vi "Send GPIB commands.vi"(0 "Command list 1":T1(array[cluster]) {"Module" items=["Atom removal 1", "Atom removal 2", "B-field off", "CMOT", "Defaults", "Final B-field ramps", "Fluorescence pulse", "High field", "High field ARP", "Loading cart QT", "Loading sci QT", "Low field", "Low field ARP", "Mol OD image", "Mol picture", "Mol probe pulse", "Molasses", "MOT off", "MOT on", "OD image", "Optical pumping", "OT B-field off", "Picture", "Probe pulse", "QT off for OT", "Quadrupole trap off", "Quadrupole trap", "Quantization axis", "S-G separation", "STIRAP back for imaging", "STIRAP", "TTL high", "TTL low", "GPIB", "Utility Module 1", "Utility Module 2", "Utility Module 3", "Utility Module 4", "Utility Module 5", "Utility Module 6", "Utility Module 7", "Utility Module 8", "Utility Module 9"]; "Abs Start Time" format="%.3f"}, 1 "End time":dbl=83073.546, 2 "Abs start time":dbl=62269.999980926514, 3 "do it!":bool=TRUE) -> ()   [LabVIEW 2017]
doc: "This sends out GPIB commands during the experiment (after the DIO (TTL) board has been triggered."
uses:
  globals/Modules global.vi
panel:
  out "Array 2":dbl[](array[numeric])
  out "Array":string[](array[string])
  out "sorted array":T1(array[cluster])
  out "total time":dbl
  out "start time":dbl=3231522488.434
  in  "timeout ms":i32=1000
  out "error out":errorcluster
  # "enabled  time                                      GPIB address                       command"
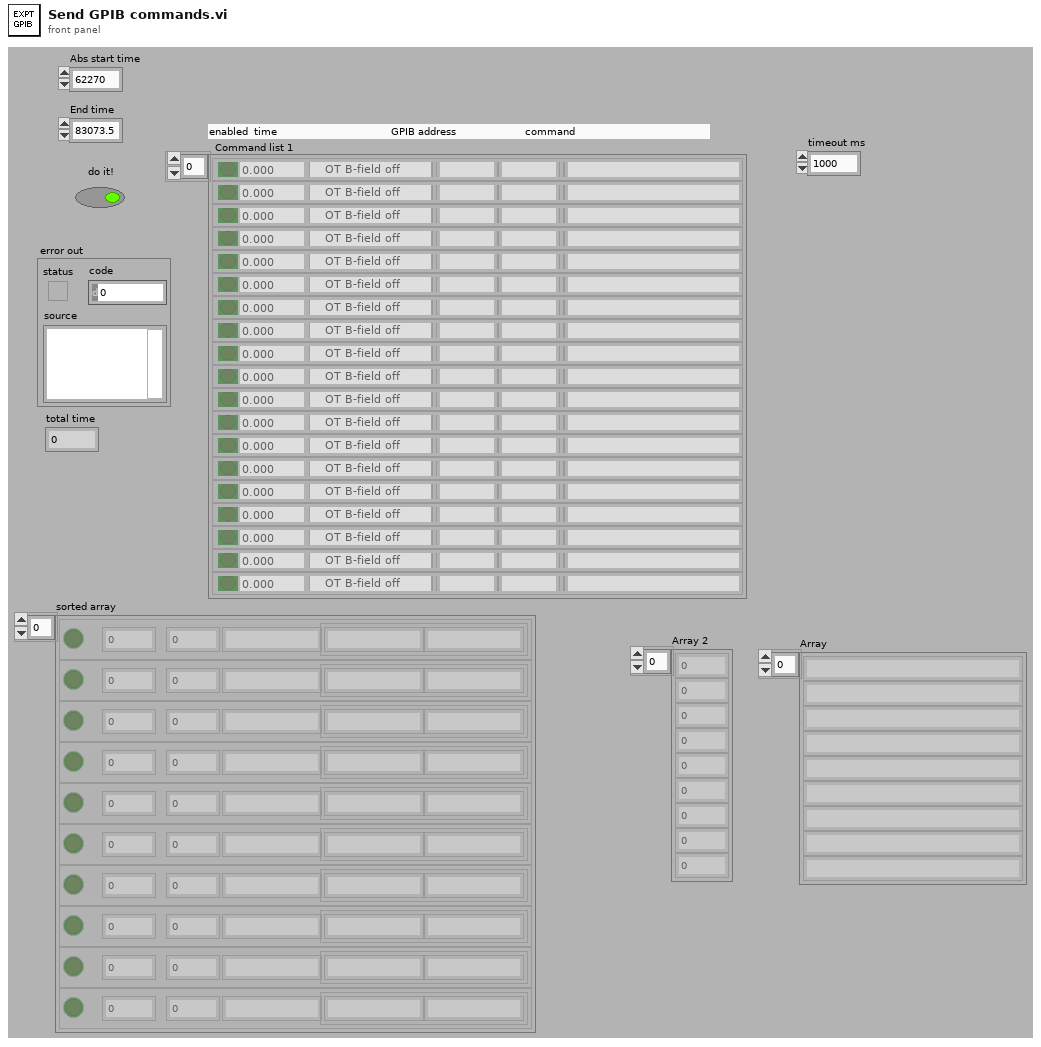
[diagram p1: front panel]
types:
  T1 = cluster{"Enable":bool, "Abs Start Time":dbl, "Module":u16, "String":string, "Array":string[]}[]
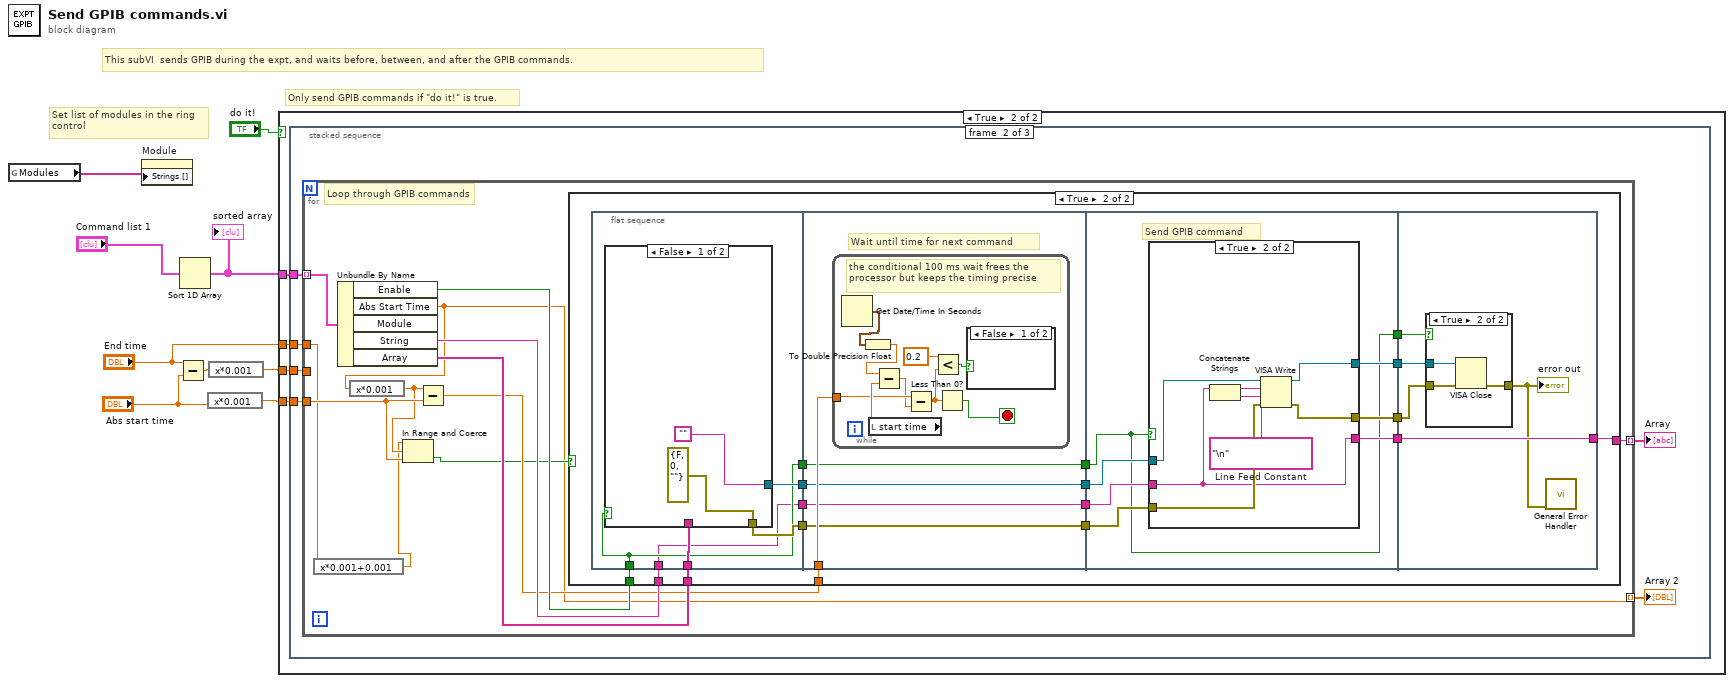
[diagram p0: block diagram]
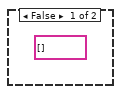
[diagram p2: hidden frame]
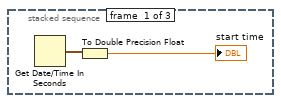
[diagram p3: hidden frame]
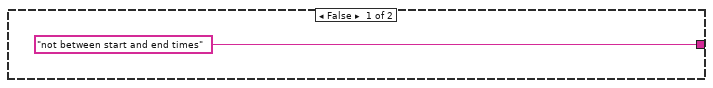
[diagram p4: hidden frame]
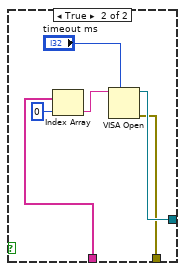
[diagram p5: hidden frame]
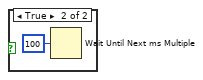
[diagram p6: hidden frame]
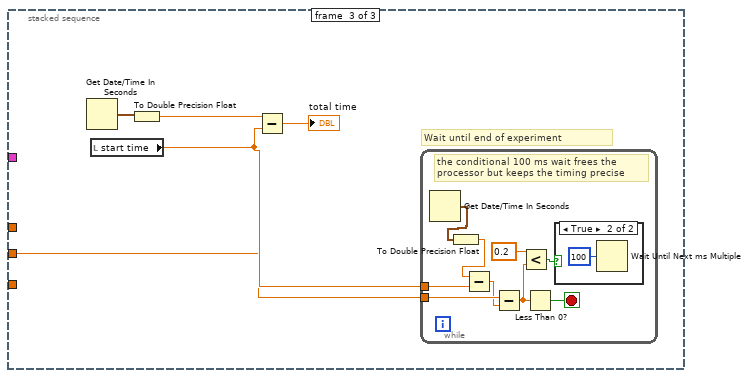
[diagram p9: hidden frame]
diagram:
  # "Set list of modules in the ring control"
  # "Only send GPIB commands if \"do it!\" is true."
  # "This subVI  sends GPIB during the expt, and waits before, between, and after the GPIB commands."
  n1 = global read "Modules global.vi" "Modules"() -> (w1:string[])
  n2 = property on="Module" class="Ring (strict)"("Strings []"=w1) -> ()  [unwired: 2 in, 2 out]
  n3 = Subtract(x="End time", y="Abs start time") -> (x-y=w8:dbl)
  n4 = Sort 1D Array(array="Command list 1") -> (sorted array=w3:T1)
  "sorted array" <- w3
  n5 = expression code="x*0.001"("Abs start time") -> (w5:dbl)
  n6 = expression code="x*0.001"(w8) -> (w7:dbl)
  n7 = case shown="True" "do it!" {
    tunnel: w5 -> [_ w13]
    tunnel: w7 -> [_ w12]
    tunnel: w3 -> [_ w11]
    tunnel: "End time" -> [_ w10]
    frame False {
      (unwired) string[] []
    }
    frame True {
      n8 = stacked-sequence {
        tunnel: w13 -> [_ w21 _]
        tunnel: w12 -> [_ w18 w106]
        tunnel: w11 -> [_ w20 _]
        tunnel: w10 -> [_ w17 _]
        frame #0 {
          n9 = Get Date/Time In Seconds() -> (seconds since 1Jan1904=w15:timestamp)
          n10 = To Double Precision Float(number=w15) -> (double precision float=→"start time":dbl)
        }
        frame #1 {
          n11 = for {
            tunnel: w20 -> [w33] mode=indexing
            tunnel: w21 -> [w27]
            tunnel: w18 -> [_]
            tunnel: [w26] -> w16 mode=indexing
            tunnel: [w22] -> w19 mode=indexing
            tunnel: w17 -> [w24]
            # "Loop through GPIB commands"
            n12 = expression code="x*0.001+0.001"(w24) -> (w23:dbl)
            n13 = Unbundle By Name(w33) -> ("Enable"=w30:bool, "Abs Start Time"=w22:dbl, "String"=w32:string, "Array"=w31:string[])  [unwired: 1 out]
            n14 = expression code="x*0.001"(w22) -> (w25:dbl)
            n15 = In Range and Coerce(upper limit=w23, x=w25, lower limit=w27) -> (In Range?=w28:bool)  [unwired: 1 out]
            n16 = Subtract(x=w25, y=w27) -> (x-y=w29:dbl)
            n17 = case shown="True" w28 {
              tunnel: w32 -> [_ w49]
              tunnel: w31 -> [_ w48]
              tunnel: w30 -> [_ w50]
              tunnel: w29 -> [_ w51]
              tunnel: ["not between start and end times" ("String") w36] -> w26
              frame False {
              }
              frame True {
                n18 = flat-sequence {
                  tunnel: w50 -> [w53]
                  tunnel: w49 -> [w52]
                  tunnel: w48 -> [w54]
                  tunnel: [w52] -> w47
                  tunnel: [w56] -> w46
                  tunnel: [w55] -> w45
                  tunnel: [w53] -> w44
                  tunnel: w51 -> [w69]
                  tunnel: w47 -> [w66]
                  tunnel: w46 -> [w67]
                  tunnel: w45 -> [w65]
                  tunnel: w44 -> [w68]
                  tunnel: [w68] -> w43
                  tunnel: [w67] -> w42
                  tunnel: [w66] -> w41
                  tunnel: [w65] -> w40
                  tunnel: w43 -> [w80]
                  tunnel: w42 -> [w84]
                  tunnel: w41 -> [w85]
                  tunnel: w40 -> [w86]
                  tunnel: [w83] -> w39
                  tunnel: [w82] -> w38
                  tunnel: [w81] -> w37
                  tunnel: [w80] -> w35
                  tunnel: w39 -> [w99]
                  tunnel: w38 -> [w100]
                  tunnel: w37 -> [w101]
                  tunnel: [w101] -> w36
                  tunnel: w35 -> [w98]
                  frame #0 {
                    n19 = case shown="False" w53 {
                      tunnel: ["" w61] -> w56
                      tunnel: [errorcluster {"status"=FALSE, "code"=0, "source"=""} ("VISA Error") w60] -> w55
                      tunnel: w54 -> [_ w59]
                      frame False {
                      }
                      frame True {
                        n20 = Index Array(array=w59, index=0) -> (element=w62:string)
                        n21 = VISA Open(timeout (0)="timeout ms", VISA resource name=w62) -> (VISA resource name=w61:refnum<visa-resource-name>, error out=w60:errorcluster)  [unwired: 3 in]
                      }
                    }
                  }
                  frame #1 {
                    # "Wait until time for next command"
                    n22 = while {
                      tunnel: w69 -> [w71]
                      stop <- w75 stop-if-true
                      # "the conditional 100 ms wait frees the processor but keeps the timing precise"
                      n23 = Get Date/Time In Seconds() -> (seconds since 1Jan1904=w74:timestamp)
                      n24 = To Double Precision Float(number=w74) -> (double precision float=w73:dbl)
                      n25 = local read "start time"() -> (w72:dbl)
                      n26 = Subtract(x=w73, y=w72) -> (x-y=w70:dbl)
                      n27 = Subtract(x=w71, y=w70) -> (x-y=w76:dbl)
                      n28 = Less?(x=0.2 ("y"), y=w76) -> (x < y?=w77:bool)
                      n29 = Less Than 0?(x=w76) -> (x < 0?=w75:bool)
                      n30 = case shown="False" w77 {
                        frame False {
                        }
                        frame True {
                          n31 = Wait Until Next ms Multiple(millisecond multiple=u32 100) -> ()  [unwired: 1 out]
                        }
                      }
                    }
                  }
                  frame #2 {
                    # "Send GPIB command"
                    n32 = case shown="True" w80 {
                      tunnel: w86 -> [w87 w95]
                      tunnel: w85 -> [w88 w92]
                      tunnel: w84 -> [w89 w96]
                      tunnel: [w89 w94] -> w83
                      tunnel: [w88 w92] -> w81
                      tunnel: [w87 w93] -> w82
                      frame False {
                      }
                      frame True {
                        w90 = "\n"  # Line Feed Constant
                        n33 = Concatenate Strings(w92, w90) -> (w91:string)
                        n34 = VISA Write(VISA resource name=w96, write buffer=w91, error in (no error)=w95) -> (VISA resource name out=w94:refnum<visa-resource-name>, error out=w93:errorcluster)  [unwired: 1 out]
                      }
                    }
                  }
                  frame #3 {
                    n35 = case shown="True" w98 {
                      tunnel: [w102 w105] -> w97
                      tunnel: w100 -> [w102 w104]
                      tunnel: w99 -> [_ w103]
                      frame False {
                      }
                      frame True {
                        n36 = VISA Close(VISA resource name=w103, error in (no error)=w104) -> (error out=w105:errorcluster)
                      }
                    }
                    "error out" <- w97
                    n37 = call <vilib>:"General Error Handler.vi"("error in (no error)"=w97) -> ()  [unwired: 10 in, 5 out]
                  }
                }
              }
            }
          }
          "Array" <- w16
          "Array 2" <- w19
        }
        frame #2 {
          # "Wait until end of experiment"
          n38 = Get Date/Time In Seconds() -> (seconds since 1Jan1904=w110:timestamp)
          n39 = local read "start time"() -> (w107:dbl)
          n40 = To Double Precision Float(number=w110) -> (double precision float=w109:dbl)
          n41 = Subtract(x=w109, y=w107) -> (x-y=→"total time":dbl)
          n42 = while {
            tunnel: w107 -> [w113]
            tunnel: w106 -> [w112]
            stop <- w116 stop-if-true
            # "the conditional 100 ms wait frees the processor but keeps the timing precise"
            n43 = Get Date/Time In Seconds() -> (seconds since 1Jan1904=w114:timestamp)
            n44 = To Double Precision Float(number=w114) -> (double precision float=w115:dbl)
            n45 = Subtract(x=w115, y=w113) -> (x-y=w111:dbl)
            n46 = Subtract(x=w112, y=w111) -> (x-y=w117:dbl)
            n47 = Less?(x=0.2 ("y"), y=w117) -> (x < y?=w118:bool)
            n48 = Less Than 0?(x=w117) -> (x < 0?=w116:bool)
            n49 = case shown="True" w118 {
              frame False {
              }
              frame True {
                n50 = Wait Until Next ms Multiple(millisecond multiple=u32 100) -> ()  [unwired: 1 out]
              }
            }
          }
        }
      }
    }
  }
